vi "pmu_Check PMU Parameter Error (Std 2011).vi"(8 "error in (no error)":errorcluster, 11 "time base":u32=10000000) -> (0 "error out":errorcluster)   [LabVIEW 2015, in "NI_EP_PMU.lvlib"]
uses:
  <vilib>/addons/Electrical Power/PMU/NI_EP_PMU.lvlib
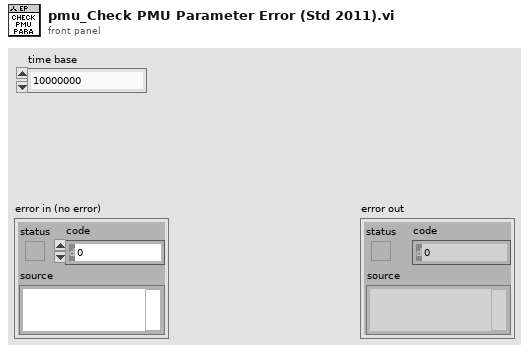
[diagram p1: front panel]
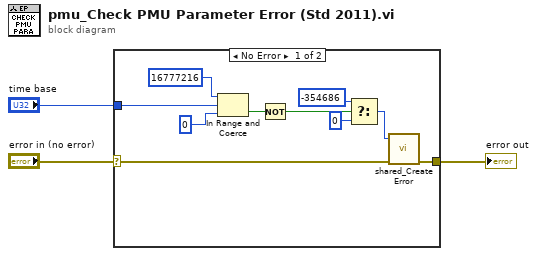
[diagram p0: block diagram]
diagram:
  n1 = case shown="No Error" "error in (no error)" {
    selector: "error in (no error)" -> [w9 w14]
    tunnel: "time base" -> [w8 _]
    tunnel: [w11 w14] -> w2
    frame No Error {
      n2 = In Range and Coerce(upper limit=u32 16777216 ("lower limit"), x=w8, lower limit=u32 0) -> (In Range?=w7:bool)  [unwired: 1 out]
      n3 = Not(x=w7) -> (.not. x?=w6:bool)
      n4 = Select(t=-354686 ("error code (0)"), s=w6, f=0 ("error code (0)")) -> (s? t:f=w10:i32)
      n5 = call <vilib>:"shared_Create Error.vi"("error in (no error)"=w9, "error code (0)"=w10) -> ("error out"=w11:errorcluster)  [unwired: 9 in]
    }
    frame Error {
    }
  }
  "error out" <- w2
